vi "Auto Shooter Mode.vi"(0 "Shooter Command":T1, 7 "Current Angle":dbl, 9 "Ball Loaded?":bool) -> (8 "Secure Ball?":bool, 10 "Angle In Range?":bool, 11 "RPM Ready?":bool, 12 "Vision Target Aligned?":bool, 13 "Intake Ready?":bool, 14 "State":T5, 15 "Shooter Ready?":bool, 16 "Left Output":dbl, 17 "Right Output":dbl, 18 "Angle Motor Output":dbl, 19 "Trigger Output":dbl)   [LabVIEW 2015]
uses:
  Common Code/Shooter State.ctl
  Common Code/Shooter Command Cluster.ctl
  Common Code/Shooter Commands.ctl
  Common Code/Shoot Modes Enum.ctl
  Common Code/Shot Type.ctl
  Common Code/Shooter Presets.ctl
  Common Code/Shot Presets.ctl
  Common Code/Intake States.ctl
  Common Code/Intake Commands.ctl
  Common Code/Change Detect Int.vi
  Common Code/Change Detect Double.vi
  Robot Global Data.vi
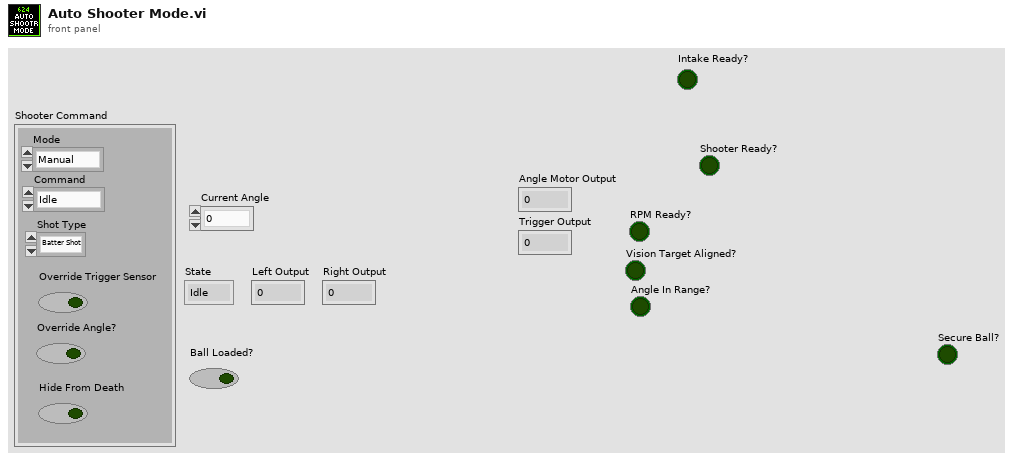
[diagram p1: front panel]
types:
  T1 = typedef "Shooter Command Cluster.ctl" = cluster{"Command":T2, "Mode":T3, "Shot Type":T4, "Override Trigger Sensor":bool, "Override Angle?":bool, "Hide From Death":bool}
  T2 = typedef "Shooter Commands.ctl" = enum16{"Idle", "Prime Shooter", "Shoot"}
  T3 = typedef "Shoot Modes Enum.ctl" = enum16{"Manual", "Safe", "Auto"}
  T4 = typedef "Shot Type.ctl" = enum16{"Batter Shot", "Corner Shot", "Cleat Shot", "Vision Shot", "Deep Middle Shot"}
  T5 = typedef "Shooter State.ctl" = enum16{"Idle", "Settle Ball", "Warmup", "Shooter Ready", "Shoot"}
  T6 = typedef "Intake Commands.ctl" = enum16{"Settle Ball", "Unload", "Load", "Pull up", "Drop low", "Idle", "Lift Half", "Go To Angle"}
  T7 = typedef "Intake States.ctl" = enum16{"Idle", "Set roller speed", "Move to angle", "Go Hard or Go Home", "Ball Settle"}
  T8 = typedef "Shooter Presets.ctl" = cluster{"Batter Shot":T9, "Deep Middle":T9, "Manual Shot":T9, "Left Ticks Per Rotation":dbl, "Right Ticks Per Rotation":dbl, "Low Bar Shot":T9, "Shooter RPM Tolerance":dbl, "Trigger Power":dbl, "Fire from Load Delay":i32, "Max Angle":dbl, "Min Angle":dbl, "Angle PID gains":cluster{"P":dbl, "I":dbl, "D":dbl}, "Angle Output":cluster{"output high":dbl, "output low":dbl}, "Shooter Angle Tolerance":dbl, "Vision Shoot x^2":dbl, "Vision Shoot x":dbl, "Feed Forward Max Accel":dbl, "Feed Forward Kv":dbl, "Backwards Trigger":dbl, "Shot Finish Delay (ms)":dbl, "Angle Max Current":dbl, "Angle Current Trip Time":dbl, "Intake Angle":dbl, "Vision Shoot c":dbl, "Reset?":bool, "Button Release Delay":dbl, "Angle Pot x":dbl, "Angle Pot c":dbl, "Ignore Angle?":bool, "Max RPM":dbl, "Safty Frist Angle":dbl, "Intake Danger Height":dbl, "Angle Pot B":i32, "Angle Pot M":dbl, "FF Finish RPM":dbl, "RPM PID Right":cluster{"P":dbl, "I":dbl, "D":dbl, "FF":dbl}, "RPM PID Left":cluster{"P":dbl, "I":dbl, "D":dbl, "FF":dbl}, "Backwards RPM":dbl, "Vision RPM":dbl, "Run Wheels Backward Delay":u32, "Cleat Shot":T9}
  T9 = typedef "Shot Presets.ctl" = cluster{"L":dbl, "R":dbl, "A":dbl}
  T10 = typedef "Dashboard Control Data.ctl" = cluster{"Shooter Presets":T8, "Encoder Control":T11, "Steer PID output":cluster{"output high":dbl, "output low":dbl}, " Steer PID gains":cluster{"proportional gain (Kc)":dbl, "integral time (Ti, min)":dbl, "derivative time (Td, min)":dbl}, "Drivetrain Settings":T12, "Vision Packet":T13, "Dashboard Drivetrain Command":T14, "Info/Command Cluster":T16, "Ball Vision Packet":T17, "Intake Presets":T19, "Intake Encoder Control":T21, "Climb Presets":T22, "Goal Output Range":cluster{"output high":dbl, "output low":dbl}, "Enabled Systems":T23, "Auton Presets":T24, "Pressure M":dbl, "Pressure B":dbl, "Vision Timeout":dbl, "Auto-Shift":T25}
  T11 = typedef "Encoder Control.ctl" = cluster{"Right Tick Constant":dbl, "Left Tick Constant":dbl, "Reset?":bool, "Y Dist":cluster{"PID gains":cluster{"proportional gain (Kc)":dbl, "integral time (Ti, min)":dbl, "derivative time (Td, min)":dbl}}, "Y Stop Thresh":dbl, "Y Stop Speed":dbl}
  T12 = typedef "Drivetrain Settings.ctl" = cluster{"Gyro Tolerance":dbl, "Throttle Ramp (ms)":dbl, "Kv":dbl, "Ka":dbl, "Feed Forward P":dbl, "Feed Forward D":dbl, "Goal Vision PID gains":cluster{"proportional gain (Kc)":dbl, "integral time (Ti, min)":dbl, "derivative time (Td, min)":dbl}, "Goal Detection Window":dbl, "Creep Rate":dbl, "Vision Throttle Threshold":dbl, "Min Turn Output":dbl, "Left Batter Angle":dbl, "Right Batter Angle":dbl}
  T13 = typedef "Goal Vision Packet.ctl" = cluster{"Distance":dbl, "Center X":dbl, "Center Y":dbl, "Found Target?":bool, "Robot Center":dbl, "Angle":dbl}
  T14 = typedef "Dashboard Drivetrain Command.ctl" = cluster{"Drivetrain Vision":T15}
  T15 = typedef "Drivetrain Vision.ctl" = cluster{"Goal Window":dbl, "Ball Window":dbl}
  T16 = typedef "Ball Tracking Command Cluster.ctl" = cluster{"Distance to Ball":dbl, "Desired Angle":dbl, "Command":enum16{"Turn to Ball", "Turn to Angle", "Get Distance"}, "Pixels from Center":dbl}
  T17 = typedef "Ball Vision Packet.ctl" = cluster{"Ball Detected?":bool, "Distance to Ball":dbl, "Desired Angle":dbl, "Pixels from Center":dbl, "Tracking mode":T18}
  T18 = typedef "Tracking Mode.ctl" = enum16{"Turn to Ball", "Turn to Angle"}
  T19 = typedef "Intake Presets.ctl" = cluster{"Intake Speed":dbl, "Outake Speed":dbl, "Low Height":dbl, "Half Height":dbl, "High Idle Height":dbl, "Angle Speed":dbl, "Angle Tolerance":dbl, "Encoder Scale":dbl, "Load Height":dbl, "Output Range":T20, "Rotation Power Max/Min":dbl, "MaxCurrent":dbl, "Intake Trip Time":dbl, "Idle Height":dbl, "Max Height":dbl, "Reset Encoders?":bool, "PID gains":cluster{"proportional gain (Kc)":dbl, "integral time (Ti, min)":dbl, "derivative time (Td, min)":dbl}, "Intake Stop Delay":u32, "Settle Time":dbl, "Settle Wait Time":dbl, "Pull Up Delay":dbl}
  T20 = typedef "Drivetrain Output Range.ctl" = cluster{"output high":dbl, "output low":dbl}
  T21 = typedef "IntakeEcoderControl.ctl" = cluster{"Arm Tick Constant":dbl, "Reset?":bool, "Y Dist":cluster{"PID gains":cluster{"proportional gain (Kc)":dbl, "integral time (Ti, min)":dbl, "derivative time (Td, min)":dbl}}, "Y Stop Thresh":dbl, "Y Stop Speed":dbl}
  T22 = typedef "Climb Presets.ctl" = cluster{"Pull Power":dbl, "Extend Power":dbl}
  T23 = typedef "Enabled Systems.ctl" = cluster{"Shoot":bool, "Intake":bool, "DT":bool, "Gyro":bool, "100ms":bool, "US":bool}
  T24 = typedef "Autonomous Presets.ctl" = cluster{"Pitch Limit":dbl, "Roll Limit":dbl, "Start Position":dbl, "Cross Position":dbl}
  T25 = typedef "Auto Shift Cluster.ctl" = cluster{"Delay":dbl, "Speed Thresh":dbl, "Upshift Accel":dbl, "Upshift Throttle":dbl, "Upshift Throttle Accel":dbl, "Downshift Throttle":dbl, "Downshift Throttle Accel":dbl}
  T26 = typedef "Intake Commands Cluster.ctl" = cluster{"Intake Commands":T6, "Intake Mode":T27, "Override IR":bool, "Angle Target":dbl}
  T27 = typedef "Intake Mode.ctl" = enum16{"Safe", "Auto", "Manual"}
  T28 = typedef "Intake Status Cluster.ctl" = cluster{"Roller Power":dbl, "Angle Power":dbl, "Intake Mode":T27, "Intake States":T7, "Rollers Active?":bool, "Current Height":dbl, "Target Height":dbl, "Encoder Raw Position":dbl, "Forward Tripped?":bool, "Backward Tripped?":bool, "Override IR?":bool}
  T29 = typedef "Shooter State Cluster.ctl" = cluster{"State":T5, "Left RPM":dbl, "Right RPM":dbl, "Shooter Ready?":bool, "Ball Loaded?":bool, "Current Angle":dbl, "Angle Motor Output":dbl, "Trigger Output":dbl, "Angle Ready?":bool, "RPM Ready?":bool, "Vision Ready?":bool, "Ball Loaded?":bool, "Mode":T3, "Shot Type":T4, "Pot Height":dbl, "Current Tripped Forward?":bool, "Current Tripped Backward?":bool, "Right Servo":i32, "Left Servo":i32, "IR Override":bool, "Intake Danger?":bool, "Intake Angle Ready?":bool}
  T30 = typedef "Drivetrain Status Cluster.ctl" = cluster{"Modes":T31, "Y (Throttle)":dbl, "X (Steer)":dbl, "Gyro In Range?":bool, "Distance Drive Finished?":bool, "Stop Eject Lockout":bool, "Dist Drive Status":T32, "Y Target":dbl, "Heading Target":dbl, "Vision Target Aligned?":bool, "Gear":dbl, "1st Gear Time":dbl, "2nd Gear Time":dbl, "1st Gear Shifts":dbl, "2nd Gear Shifts":dbl}
  T31 = typedef "Drivetrain Modes.ctl" = enum16{"Tank", "Climb", "Manual", "Goal Vision Targeting", "PID Distance Drive", "Hybrid", "Gyro Steer"}
  T32 = typedef "Dist Drive Status.ctl" = cluster{"Y In Range":bool, "X In Range":bool, "Gyro In Range":bool, "Y Dist":dbl, "X Dist":dbl, "Gyro":dbl}
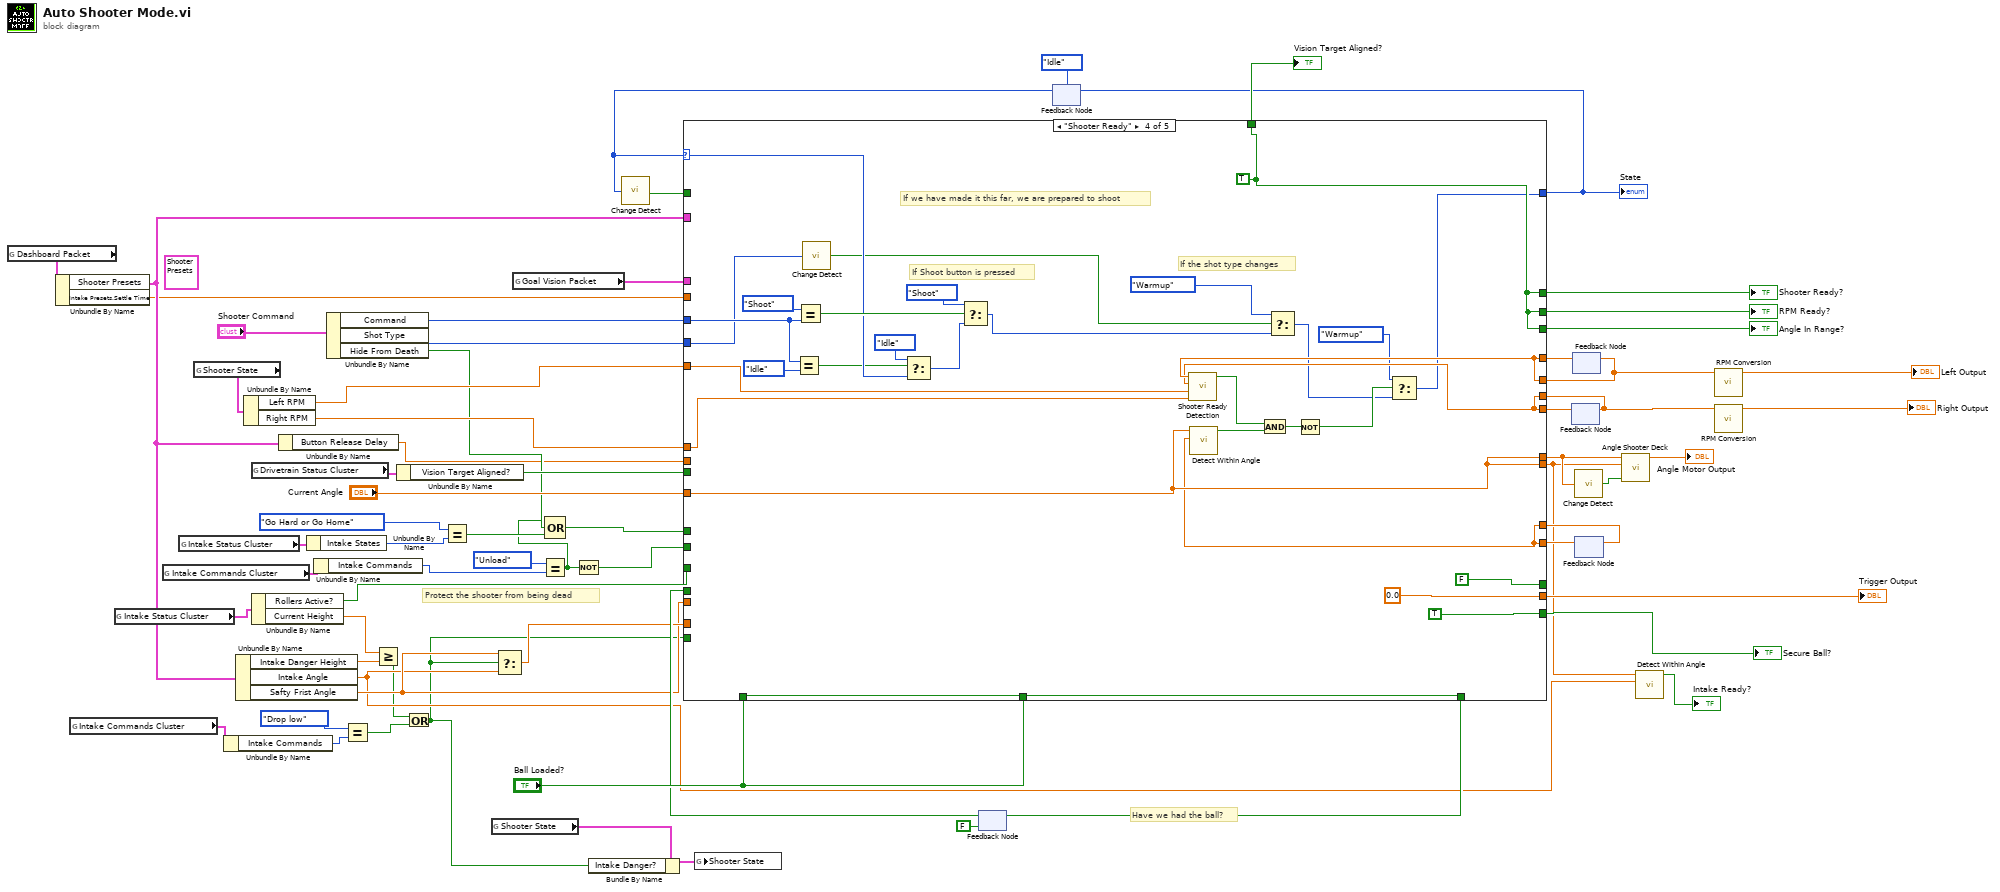
[diagram p0: block diagram]
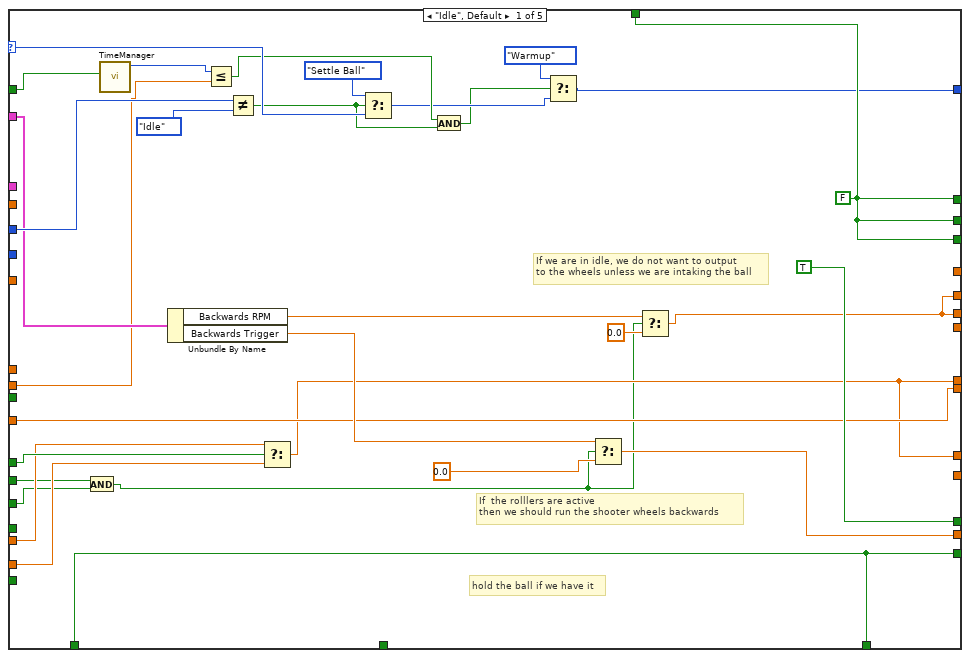
[diagram p2: hidden frame]
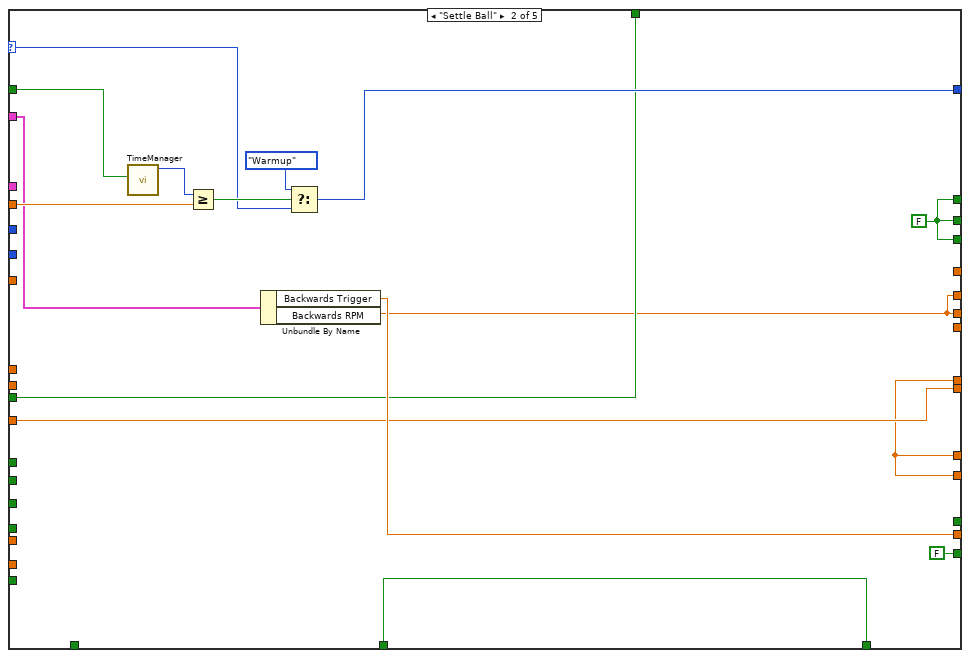
[diagram p3: hidden frame]
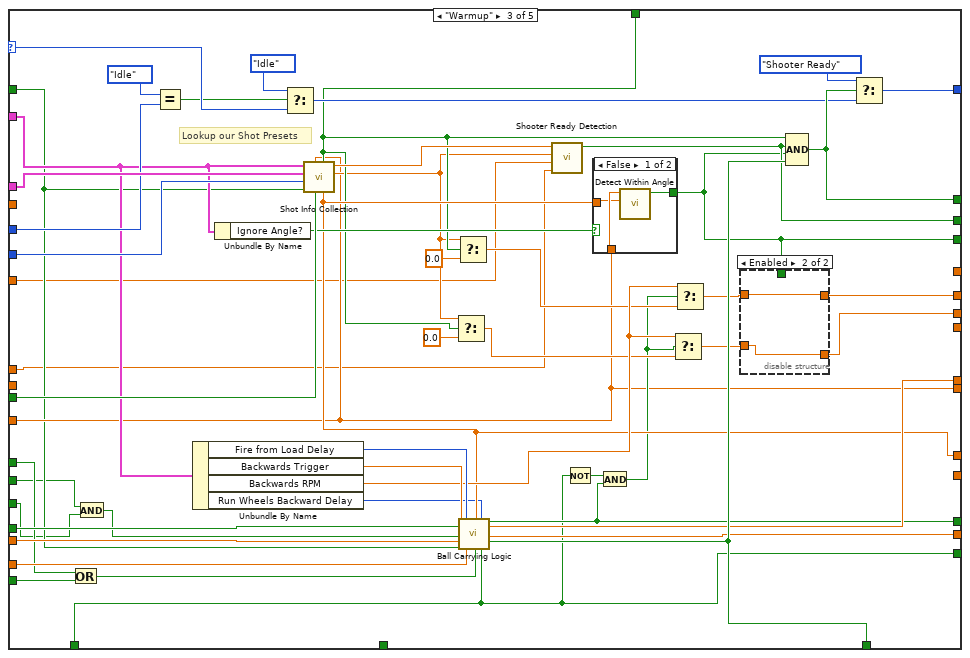
[diagram p4: hidden frame]
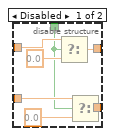
[diagram p5: hidden frame]
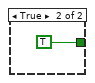
[diagram p6: hidden frame]
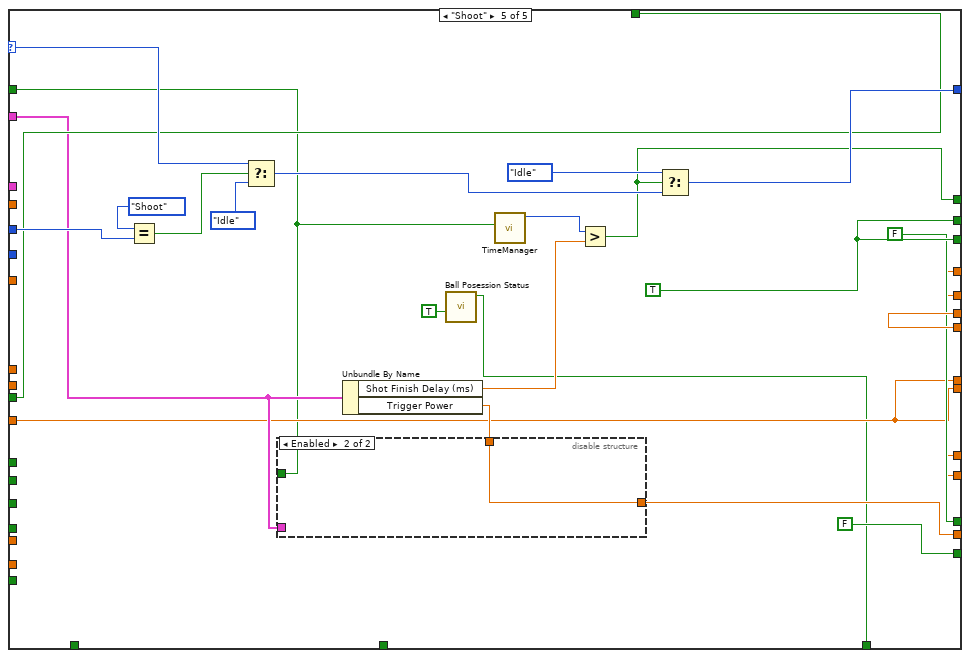
[diagram p7: hidden frame]
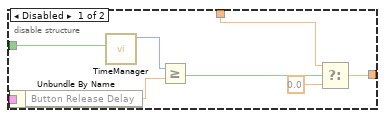
[diagram p8: hidden frame]
diagram:
  (unwired) T8 {"Batter Shot"={"L"=0.0, "R"=0.0, "A"=0.0}, "Deep Middle"={"L"=0.0, "R"=0.0, "A"=0.0}, "Manual Shot"={"L"=0.0, "R"=0.0, "A"=0.0}, "Left Ticks Per Rotation"=0.0, "Right Ticks Per Rotation"=0.0, "Low Bar Shot"={"L"=0.0, "R"=0.0, "A"=0.0}, "Shooter RPM Tolerance"=0.0, "Trigger Power"=0.0, "Fire from Load Delay"=0, "Max Angle"=0.0, "Min Angle"=0.0, "Angle PID gains"={"P"=1.0, "I"=0.01, "D"=0.0}, "Angle Output"={"output high"=1.0, "output low"=-1.0}, "Shooter Angle Tolerance"=0.0, "Vision Shoot x^2"=0.0, "Vision Shoot x"=0.0, "Feed Forward Max Accel"=0.0, "Feed Forward Kv"=0.0, "Backwards Trigger"=0.0, "Shot Finish Delay (ms)"=0.0, "Angle Max Current"=0.0, "Angle Current Trip Time"=0.0, "Intake Angle"=0.0, "Vision Shoot c"=0.0, "Reset?"=FALSE, "Button Release Delay"=0.0, "Angle Pot x"=0.0, "Angle Pot c"=0.0, "Ignore Angle?"=FALSE, "Max RPM"=0.0, "Safty Frist Angle"=0.0, "Intake Danger Height"=0.0, "Angle Pot B"=0, "Angle Pot M"=0.0, "FF Finish RPM"=0.0, "RPM PID Right"={"P"=1.0, "I"=0.01, "D"=0.0, "FF"=0.0}, "RPM PID Left"={"P"=1.0, "I"=0.01, "D"=0.0, "FF"=0.0}, "Backwards RPM"=0.0, "Vision RPM"=0.0, "Run Wheels Backward Delay"=0, "Cleat Shot"={"L"=0.0, "R"=0.0, "A"=0.0}} ("Shooter Presets")
  # "Protect the shooter from being dead"
  # "Have we had the ball?"
  n1 = global read "Robot Global Data.vi" "Dashboard Packet"() -> (w48:T10)
  n2 = Unbundle By Name(w48) -> ("Shooter Presets"=w14:T8, "Intake Presets.Settle Time"=w8:dbl)
  n3 = global read "Robot Global Data.vi" "Intake Commands Cluster"() -> (w20:T26)
  n4 = global read "Robot Global Data.vi" "Intake Status Cluster"() -> (w47:T28)
  n5 = global read "Robot Global Data.vi" "Intake Commands Cluster"() -> (w7:T26)
  n6 = global read "Robot Global Data.vi" "Intake Status Cluster"() -> (w25:T28)
  n7 = global read "Robot Global Data.vi" "Shooter State"() -> (w39:T29)
  n8 = Unbundle By Name(w20) -> ("Intake Commands"=w19:T6)
  n9 = Unbundle By Name(w14) -> ("Intake Danger Height"=w44:dbl, "Intake Angle"=w27:dbl, "Safty Frist Angle"=w42:dbl)
  n10 = Unbundle By Name(w39) -> ("Left RPM"=w38:dbl, "Right RPM"=w37:dbl)
  n11 = global read "Robot Global Data.vi" "Drivetrain Status Cluster"() -> (w62:T30)
  n12 = Unbundle By Name(w47) -> ("Rollers Active?"=w60:bool, "Current Height"=w45:dbl)
  n13 = Unbundle By Name(w14) -> ("Button Release Delay"=w3:dbl)
  n14 = Unbundle By Name(w25) -> ("Intake States"=w2:T7)
  n15 = Unbundle By Name(w7) -> ("Intake Commands"=w6:T6)
  n16 = Unbundle By Name("Shooter Command") -> ("Command"=w67:T2, "Shot Type"=w65:T4, "Hide From Death"=w22:bool)
  n17 = Equal?(x=Intake_Commands."Drop low", y=w19) -> (x = y?=w17:bool)
  n18 = Greater Or Equal?(x=w45, y=w44) -> (x >= y?=w16:bool)
  n19 = Unbundle By Name(w62) -> ("Vision Target Aligned?"=w61:bool)
  n20 = Or(x=w16, y=w17) -> (x .or. y?=w15:bool)
  n21 = Equal?(x=Intake_States."Go Hard or Go Home", y=w2) -> (x = y?=w23:bool)
  n22 = global read "Robot Global Data.vi" "Shooter State"() -> (w32:T29)
  n23 = Select(t=w42, s=w15, f=w27) -> (s? t:f=w43:dbl)
  n24 = global read "Robot Global Data.vi" "Goal Vision Packet"() -> (w11:T13)
  n25 = Equal?(x=Intake_Commands."Unload", y=w6) -> (x = y?=w1:bool)
  n26 = Compound Arithmetic op=OR(w1, w22, w23) -> (w21:bool)
  n27 = Not(x=w1) -> (.not. x?=w4:bool)
  n28 = Bundle By Name(cluster=w32, "Intake Danger?"=w15) -> (w31:T29)
  n29 = global write "Robot Global Data.vi" "Shooter State"(w31) -> ()
  n30 = feedback #1(FALSE ("Ball Loaded?")) -> (w57:bool)
  n31 = feedback #2(Shooter_State."Idle") -> (w55:T5)
  n32 = call-poly "Change Detect.vi"("In"=w55) -> ("Changed?"=w54:bool)
  n33 = feedback #3() -> (w63:dbl)  [unwired: 1 in]
  n34 = feedback #4() -> (w64:dbl)  [unwired: 1 in]
  n35 = feedback #5() -> (w29:dbl)  [unwired: 1 in]
  n36 = case shown="\"Shooter Ready\"" w55 {
    selector: w55 -> [w95 w110 w158 w201 w232]
    tunnel: w67 -> [w96 _ w155 w208 w235]
    tunnel: [w68 w108 w118 w184 w228] -> w9
    tunnel: w14 -> [w88 w107 w146 _ w220]
    tunnel: w65 -> [_ _ w166 w181 _]
    tunnel: [w84 w101 w124 w193 w231] -> w13
    tunnel: [w84 w101 w126 w194 w215] -> w12
    tunnel: w64 -> [_ _ _ w194 w215]
    tunnel: w63 -> [_ _ _ w193 w231]
    tunnel: w38 -> [_ _ w119 w183 _]
    tunnel: w37 -> [_ _ w120 w182 _]
    tunnel: w61 -> [_ w103 w162 _ w225]
    tunnel: "Ball Loaded?" -> [_ w102 _ _ _]
    tunnel: w11 -> [_ _ w164 _ _]
    tunnel: [w80 w99 w150 w192 w216] -> w34
    tunnel: w60 -> [w78 _ w116 _ _]
    tunnel: [w92 w104 w151 0.0 ("f") w218] -> w40
    tunnel: "Ball Loaded?" -> [w87 _ w141 w207 _]
    tunnel: [w87 w102 w161 w207 w213] -> w58
    tunnel: w57 -> [_ _ w140 _ _]
    tunnel: w54 -> [w75 w114 w121 _ w214]
    tunnel: "Current Angle" -> [w90 w100 w122 w192 w216]
    tunnel: [w89 w106 w163 w197 w221] -> w52
    tunnel: [w89 w106 w123 w197 w226] -> w51
    tunnel: [w89 w106 w152 w197 w226] -> w50
    tunnel: [w89 w103 w138 w197 w225] -> w49
    tunnel: [TRUE _ w144 FALSE FALSE] -> _
    tunnel: w43 -> [w81 _ w149 _ _]
    tunnel: [w87 FALSE ("Intake High Angle Allowed?") w141 TRUE ("Intake High Angle Allowed?") FALSE ("Intake High Angle Allowed?")] -> w46
    tunnel: w15 -> [_ _ w130 _ _]
    tunnel: w42 -> [w82 _ w147 _ _]
    tunnel: [w90 w100 w122 w192 w216] -> w28
    tunnel: [w80 w99 w139 w191 w211] -> w30
    tunnel: w29 -> [_ w99 _ w191 w211]
    tunnel: w21 -> [w83 _ w131 _ _]
    tunnel: w8 -> [_ w112 _ _ _]
    tunnel: w4 -> [w79 _ w117 _ _]
    tunnel: w3 -> [w73 _ _ _ _]
    frame "Idle", Default {
      w89 = FALSE ("Shooter Ready?")
      # "hold the ball if we have it"
      # "If  the rolllers are active\nthen we should run the shooter wheels backwards"
      # "If we are in idle, we do not want to output\nto the wheels unless we are intaking the ball"
      n37 = And(x=w79, y=w78) -> (x .and. y?=w77:bool)
      n38 = call "TimeManager.vi"("Reset?"=w75) -> ("Time Since Reset"=w74:u32)  [unwired: 9 in, 1 out]
      n39 = Unbundle By Name(w88) -> ("Backwards RPM"=w85:dbl, "Backwards Trigger"=w93:dbl)
      n40 = Less Or Equal?(x=w74, y=w73) -> (x <= y?=w72:bool)
      n41 = Not Equal?(x=w96, y=Shooter_Commands."Idle" ("Command")) -> (x != y?=w76:bool)
      n42 = Select(t=w82, s=w83, f=w81) -> (s? t:f=w80:dbl)
      n43 = Select(t=Shooter_State."Settle Ball", s=w76, f=w95) -> (s? t:f=w71:T5)
      n44 = And(x=w72, y=w76) -> (x .and. y?=w70:bool)
      n45 = Select(t=Shooter_State."Warmup", s=w70, f=w71) -> (s? t:f=w68:T5)
      n46 = Select(t=w93, s=w77, f=0.0) -> (s? t:f=w92:dbl)
      n47 = Select(t=w85, s=w77, f=0.0) -> (s? t:f=w84:dbl)
    }
    frame "Settle Ball" {
      w106 = FALSE ("Vision Target Aligned?")
      n48 = call "TimeManager.vi"("Reset?"=w114) -> ("Time Since Reset"=w113:u32)  [unwired: 9 in, 1 out]
      n49 = Greater Or Equal?(x=w113, y=w112) -> (x >= y?=w111:bool)
      n50 = Unbundle By Name(w107) -> ("Backwards Trigger"=w104:dbl, "Backwards RPM"=w101:dbl)
      n51 = Select(t=Shooter_State."Warmup", s=w111, f=w110) -> (s? t:f=w108:T5)
    }
    frame "Warmup" {
      # "Lookup our Shot Presets"
      n52 = Or(x=w131, y=w130) -> (x .or. y?=w129:bool)
      n53 = And(x=w117, y=w116) -> (x .and. y?=w115:bool)
      n54 = Equal?(x=Shooter_Commands."Idle" ("y"), y=w155) -> (x = y?=w156:bool)
      n55 = Unbundle By Name(w146) -> ("Fire from Load Delay"=w160:i32, "Backwards Trigger"=w159:dbl, "Backwards RPM"=w143:dbl, "Run Wheels Backward Delay"=w132:u32)
      n56 = Unbundle By Name(w146) -> ("Ignore Angle?"=w148:bool)
      n57 = Select(t=Shooter_State."Idle", s=w156, f=w158) -> (s? t:f=w157:T5)
      n58 = call "Shot Info Collection.vi"("Vision Target Aligned? in"=w162, "Current Angle"=w122, "Reinit?"=w121, "Shot Type"=w166, "Vision Packet"=w164, "Shooter Presets"=w146) -> ("Right Wheel RPM"=w136:dbl, "Left Wheel RPM"=w142:dbl, "Angle"=w139:dbl, "Vision Target Aligned? out"=w138:bool)  [unwired: 2 in]
      n59 = Select(t=w136, s=w138, f=0.0) -> (s? t:f=w134:dbl)
      n60 = Select(t=w136, s=w138, f=0.0) -> (s? t:f=w133:dbl)
      n61 = call "Ball Carrying Logic.vi"("Backwards Trigger"=w159, "Had Ball Before?"=w140, "Rollers Active? in"=w115, "Safty Frist Angle"=w147, "Warmup Initiation"=w121, "Fire from Load Delay"=w160, "Intake Angle"=w149, "Angle in"=w139, "Intake at Dangerous Height?"=w129, "Roll Backward Delay"=w132, "Ball Loaded? in"=w141) -> ("Rollers Active? out"=w144:bool, "Angle out"=w150:dbl, "Trigger Out"=w151:dbl, "Ball Loaded? out"=w161:bool)  [unwired: 5 in]
      n62 = call "Shooter Ready Detection.vi"("Right RPM"=w120, "Left RPM"=w119, "Right RPM Target"=w136, "Left RPM Target"=w142) -> ("Shooter Ready?"=w152:bool)  [unwired: 7 in]
      n63 = Not(x=w141) -> (.not. x?=w145:bool)
      n64 = case shown="False" w148 {
        tunnel: [w178 TRUE ("In Range?")] -> w123
        tunnel: w122 -> [w177 _]
        tunnel: w139 -> [w176 _]
        frame False {
          n65 = call "Detect Within Angle.vi"("Angle Target"=w176, "Current Angle"=w177) -> ("In Range?"=w178:bool)  [unwired: 9 in]
        }
        frame True {
        }
      }
      n66 = And(x=w145, y=w144) -> (x .and. y?=w128:bool)
      n67 = Select(t=w143, s=w128, f=w134) -> (s? t:f=w125:dbl)
      n68 = Select(t=w143, s=w128, f=w133) -> (s? t:f=w127:dbl)
      n69 = disable-structure shown="Enabled" {
        disable-tunnel: w127 -> [w172 w175]
        disable-tunnel: [w171 w175] -> w126
        disable-tunnel: w125 -> [w169 w174]
        disable-tunnel: [w168 w174] -> w124
        disable-tunnel: w123 -> [w167 _]
        frame Disabled {
          n70 = Select(t=w172, s=w167, f=0.0) -> (s? t:f=w171:dbl)
          n71 = Select(t=w169, s=w167, f=0.0) -> (s? t:f=w168:dbl)
        }
        frame Enabled {
        }
      }
      n72 = Compound Arithmetic op=AND(w138, w152, w123, w161) -> (w163:bool)
      n73 = Select(t=Shooter_State."Shooter Ready", s=w163, f=w157) -> (s? t:f=w118:T5)
    }
    frame "Shooter Ready" {
      w197 = TRUE ("Vision Target Aligned?")
      # "If the shot type changes"
      # "If Shoot button is pressed"
      # "If we have made it this far, we are prepared to shoot"
      n74 = Equal?(x=w208, y=Shooter_Commands."Idle") -> (x = y?=w200:bool)
      n75 = Equal?(x=Shooter_Commands."Shoot", y=w208) -> (x = y?=w206:bool)
      n76 = call-poly "Change Detect.vi"("In"=w181) -> ("Changed?"=w180:bool)
      n77 = Select(t=Shooter_State."Idle", s=w200, f=w201) -> (s? t:f=w202:T5)
      n78 = Select(t=Shooter_State."Shoot", s=w206, f=w202) -> (s? t:f=w204:T5)
      n79 = call "Shooter Ready Detection.vi"("Right RPM"=w182, "Left RPM"=w183, "Right RPM Target"=w193, "Left RPM Target"=w194) -> ("Shooter Ready?"=w189:bool)  [unwired: 7 in]
      n80 = call "Detect Within Angle.vi"("Angle Target"=w191, "Current Angle"=w192) -> ("In Range?"=w190:bool)  [unwired: 9 in]
      n81 = And(x=w189, y=w190) -> (x .and. y?=w188:bool)
      n82 = Select(t=Shooter_State."Warmup", s=w180, f=w204) -> (s? t:f=w186:T5)
      n83 = Not(x=w188) -> (.not. x?=w187:bool)
      n84 = Select(t=Shooter_State."Warmup", s=w187, f=w186) -> (s? t:f=w184:T5)
    }
    frame "Shoot" {
      w226 = TRUE ("Vision Target Aligned?")
      n85 = Equal?(x=Shooter_Commands."Shoot", y=w235) -> (x = y?=w233:bool)
      n86 = Select(t=w232, s=w233, f=Shooter_State."Idle") -> (s? t:f=w229:T5)
      n87 = Unbundle By Name(w220) -> ("Shot Finish Delay (ms)"=w223:dbl, "Trigger Power"=w219:dbl)
      n88 = disable-structure shown="Enabled" {
        disable-tunnel: w220 -> [w243 _]
        disable-tunnel: w219 -> [w239 w244]
        disable-tunnel: [w237 w244] -> w218
        disable-tunnel: w214 -> [w236 _]
        frame Disabled {
          n89 = Unbundle By Name(w243) -> ("Button Release Delay"=w242:dbl)
          n90 = call "TimeManager.vi"("Reset?"=w236) -> ("Time Since Reset"=w241:u32)  [unwired: 9 in, 1 out]
          n91 = Greater Or Equal?(x=w241, y=w242) -> (x >= y?=w240:bool)
          n92 = Select(t=w239, s=w240, f=0.0) -> (s? t:f=w237:dbl)
        }
        frame Enabled {
        }
      }
      n93 = call "Ball Posession Status.vi"("Logical Exit?"=TRUE) -> ("Ball Posessed?"=w213:bool)  [unwired: 10 in]
      n94 = call "TimeManager.vi"("Reset?"=w214) -> ("Time Since Reset"=w222:u32)  [unwired: 9 in, 1 out]
      n95 = Greater?(x=w222, y=w223) -> (0:w221:bool)
      n96 = Select(t=Shooter_State."Idle" ("f"), s=w221, f=w229) -> (s? t:f=w228:T5)
    }
  }
  "State" <- w9
  "Trigger Output" <- w40
  "Shooter Ready?" <- w52
  "RPM Ready?" <- w50
  "Angle In Range?" <- w51
  "Vision Target Aligned?" <- w49
  "Secure Ball?" <- w46
  n97 = feedback-in #1(w58) -> ()
  n98 = feedback-in #2(w9) -> ()
  n99 = feedback-in #3(w13) -> ()
  n100 = feedback-in #4(w12) -> ()
  n101 = call-poly "Change Detect.vi"("In"=w34) -> ("Changed?"=w33:bool)
  n102 = feedback-in #5(w30) -> ()
  n103 = call "Angle Shooter Deck.vi"("reinitialize? (F)"=w33, "Shooter Angle"=w28, "Target Angle"=w34) -> ("Angle Motor Power Out"=→"Angle Motor Output":dbl)  [unwired: 8 in]
  n104 = call "Detect Within Angle.vi"("Angle Target"=w27, "Current Angle"=w28) -> ("In Range?"=→"Intake Ready?":bool)  [unwired: 9 in]
  n105 = call "RPM Conversion.vi"("RPM"=w12) -> ("RPM Out"=→"Left Output":dbl)  [unwired: 10 in]
  n106 = call "RPM Conversion.vi"("RPM"=w13) -> ("RPM Out"=→"Right Output":dbl)  [unwired: 10 in]
